vi "Close Backpressure Reader.vi"(8 "error in (no error)":errorcluster, 11 "CIPC BP References in":T1) -> (0 "error out":errorcluster)   [LabVIEW 2021, in "CIF_NI_CIPC.lvlib"]
doc: "Close the reference to the buffer without destroying the buffer."
uses:
  TypeDefs/Backpressure References.ctl
  CIF_NI_CIPC.lvlib
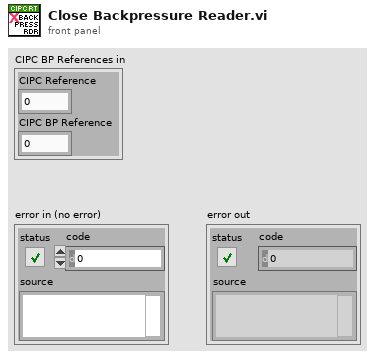
[diagram p1: front panel]
types:
  T1 = typedef "CIF_NI_CIPC.lvlib/Backpressure References.ctl" = cluster{"CIPC Reference":u64, "CIPC BP Reference":u64}
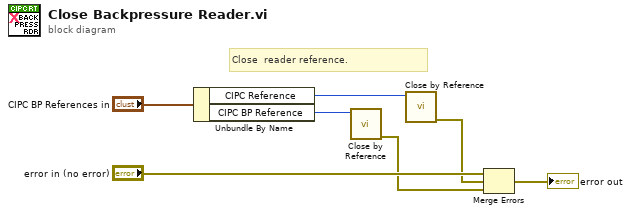
[diagram p0: block diagram]
diagram:
  # "Close  reader reference."
  n1 = Unbundle By Name("CIPC BP References in") -> ("CIPC Reference"=w4:u64, "CIPC BP Reference"=w2:u64)
  n2 = call "Close by Reference.vi"("CIPC Reference"=w2) -> ("error out"=w1:errorcluster)  [unwired: 10 in]
  n3 = call "Close by Reference.vi"("CIPC Reference"=w4) -> ("error out"=w3:errorcluster)  [unwired: 10 in]
  n4 = Merge Errors("error in (no error)", w3, w1) -> (→"error out":errorcluster)
